vi "DOConfigureCustomaPattern.vi"(0 "object in":refnum<class "AD2_DO_SDK.lvclass">, 2 "?":T1={"DO Trigger"={"secRun(0=Cont)"=0.0, "secWait"=0.0, "cRepeat(0=inf)"=0, "Repeat Trigger"=FALSE, "TrigrSrc"=enum."trigrsrcNone"}, "CustomData"=[{"Data"=[FALSE, TRUE, FALSE, FALSE, FALSE, FALSE, FALSE, FALSE, FALSE, FALSE, FALSE, FALSE, FALSE, FALSE, FALSE, FALSE, FALSE, FALSE, FALSE, FALSE, FALSE, FALSE], "Freq"=1000.0, "#Bits"=100, "Enable"=FALSE, "IdleState"=0}, {"Data"=[TRUE, TRUE, TRUE, TRUE, TRUE, FALSE, FALSE, FALSE, FALSE, FALSE, FALSE, FALSE, FALSE, FALSE, FALSE, FALSE, FALSE, FALSE, FALSE, FALSE, FALSE, FALSE], "Freq"=1000.0, "#Bits"=100, "Enable"=FALSE, "IdleState"=0}, {"Data"=[], "Freq"=0.0, "#Bits"=0, "Enable"=FALSE, "IdleState"=0}, {"Data"=[FALSE, FALSE, FALSE, FALSE, FALSE, FALSE, FALSE, FALSE, FALSE, FALSE, FALSE, FALSE, FALSE, FALSE, FALSE, FALSE, FALSE, FALSE, FALSE, FALSE, FALSE, FALSE, FALSE], "Freq"=0.0, "#Bits"=0, "Enable"=FALSE, "IdleState"=0}, {"Data"=[], "Freq"=0.0, "#Bits"=0, "Enable"=FALSE, "IdleState"=0}, {"Data"=[], "Freq"=0.0, "#Bits"=0, "Enable"=FALSE, "IdleState"=0}, {"Data"=[], "Freq"=0.0, "#Bits"=0, "Enable"=FALSE, "IdleState"=0}, {"Data"=[], "Freq"=0.0, "#Bits"=0, "Enable"=FALSE, "IdleState"=0}, {"Data"=[], "Freq"=0.0, "#Bits"=0, "Enable"=FALSE, "IdleState"=0}, {"Data"=[], "Freq"=0.0, "#Bits"=0, "Enable"=FALSE, "IdleState"=0}, {"Data"=[], "Freq"=0.0, "#Bits"=0, "Enable"=FALSE, "IdleState"=0}, {"Data"=[], "Freq"=0.0, "#Bits"=0, "Enable"=FALSE, "IdleState"=0}, {"Data"=[], "Freq"=0.0, "#Bits"=0, "Enable"=FALSE, "IdleState"=0}, {"Data"=[], "Freq"=0.0, "#Bits"=0, "Enable"=FALSE, "IdleState"=0}, {"Data"=[], "Freq"=0.0, "#Bits"=0, "Enable"=FALSE, "IdleState"=0}, {"Data"=[FALSE, FALSE, FALSE, FALSE, FALSE, FALSE, FALSE, FALSE, FALSE, FALSE, FALSE, FALSE, FALSE, FALSE, FALSE, FALSE, FALSE, FALSE, FALSE, FALSE, FALSE, FALSE, FALSE], "Freq"=0.0, "#Bits"=0, "Enable"=FALSE, "IdleState"=0}, {"Data"=[FALSE, FALSE, FALSE, FALSE, FALSE, FALSE, FALSE, FALSE, FALSE, FALSE, FALSE, FALSE, FALSE, FALSE, FALSE, FALSE, FALSE, FALSE, FALSE, FALSE, FALSE, FALSE, FALSE], "Freq"=0.0, "#Bits"=0, "Enable"=FALSE, "IdleState"=0}]}, 5 "error in (no error)":errorcluster) -> (14 "object out":refnum<class "AD2_DO_SDK.lvclass">, 19 "error out":errorcluster)   [LabVIEW 2021, in "AD2_DO_SDK.lvclass"]
uses:
  AD2_DO_SDK.lvclass
  DOConfigureCustomData.ctl
  DOTrigger.ctl
  AD2_WFG_SDK_class/AD2TriggerSources.ctl
  DOCustomData.ctl
  AD2_DO_SDK.lvclass/AD2_DO_SDK.ctl
  Olasdwf/Olasdwf.lvlib
  AD2_SDK_class/AD2_SDK.lvclass
panel:
  out "In Range?":bool
  out "pcountOfBitsMax out":u32
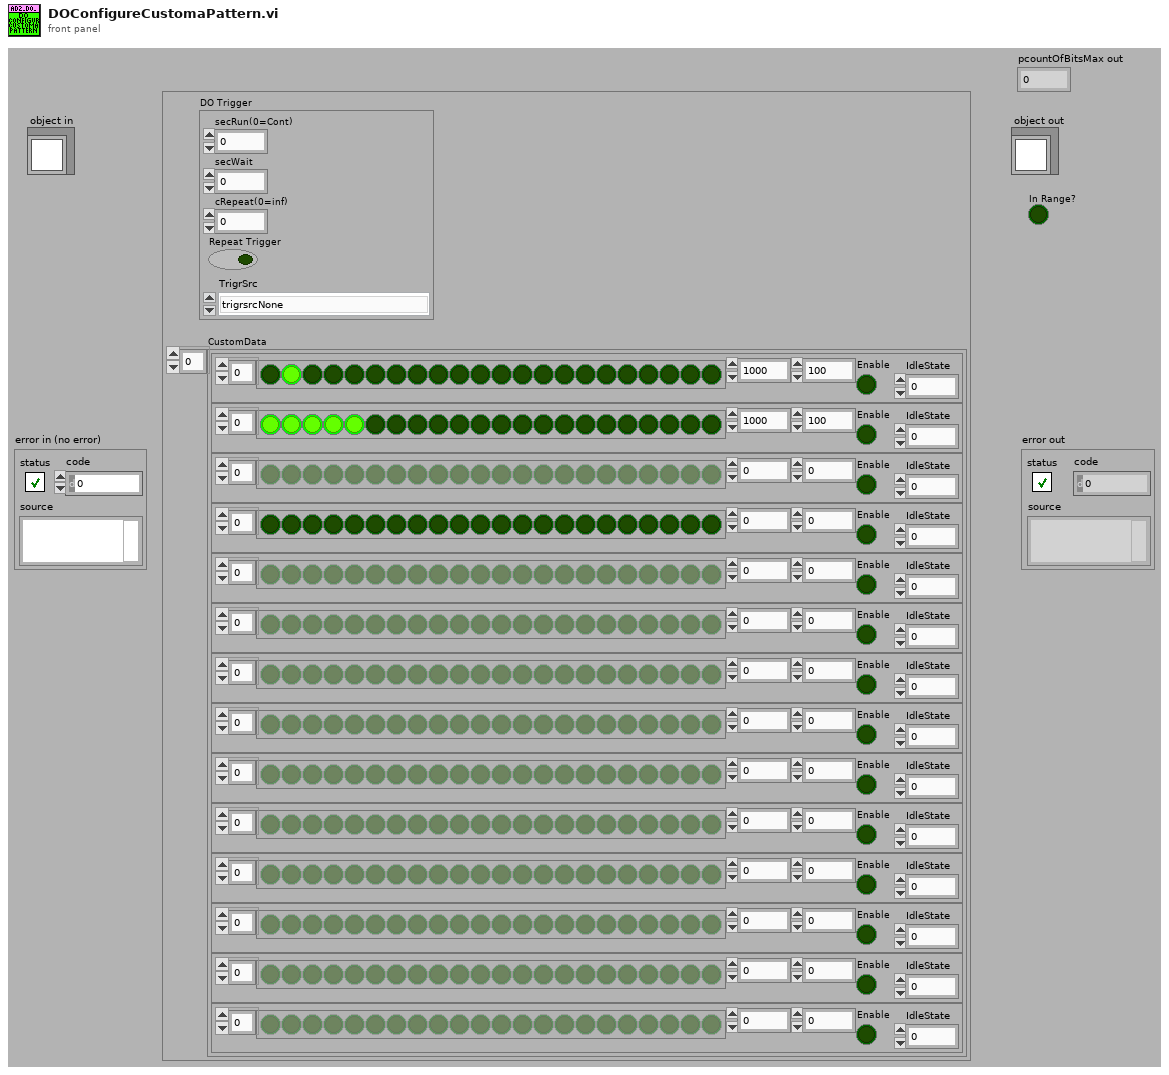
[diagram p1: front panel]
types:
  T1 = typedef "DOConfigureCustomData.ctl" = cluster{"DO Trigger":T2, "CustomData":T4}
  T2 = typedef "AD2_DO_SDK.lvclass/DOTrigger.ctl" = cluster{"secRun(0=Cont)":dbl, "secWait":dbl, "cRepeat(0=inf)":i32, "Repeat Trigger":bool, "TrigrSrc":T3}
  T3 = typedef "AD2_SDK.lvclass/AD2TriggerSources.ctl" = enum8{"trigrsrcNone", "trigsrcPC", "trigsrcDetectorAnalogIn", "trigsrcDetectorDigitalIn", "trigsrcAnalogIn", "trigsrcDigitalIn", "trigsrcDigitalOut", "trigsrcAnalogOut1", "trigsrcAnalogOut2", "trigsrcAnalogOut3", "trigsrcAnalogOut4", "trigsrcExternal1", "trigsrcExternal2", "trigsrcExternal3", "trigsrcExternal4", ""}
  T4 = typedef "AD2_DO_SDK.lvclass/DOCustomData.ctl" = cluster{"Data":bool[], "Freq":dbl, "#Bits":u32, "Enable":bool, "IdleState":u16}[]
  T5 = cluster{"NoHighBits":u32, "NoLowBits":u32, "NoInitialBits":u32, "Start High":bool}
  T6 = typedef "AD2_DO_SDK.lvclass/DOSingleCh.ctl" = cluster{"Ch Index":i32, "Enable":bool, "Clock DIvider":u32, "Type":i32, "DigitalOutOutput":u16, "IdleState":u16, "CounterData":cluster{"NoHighBits":u32, "NoLowBits":u32, "NoInitialBits":u32, "Start High":bool}, "Custom Data":cluster{"countOfBits":u32, "rgBits":u8[]}}
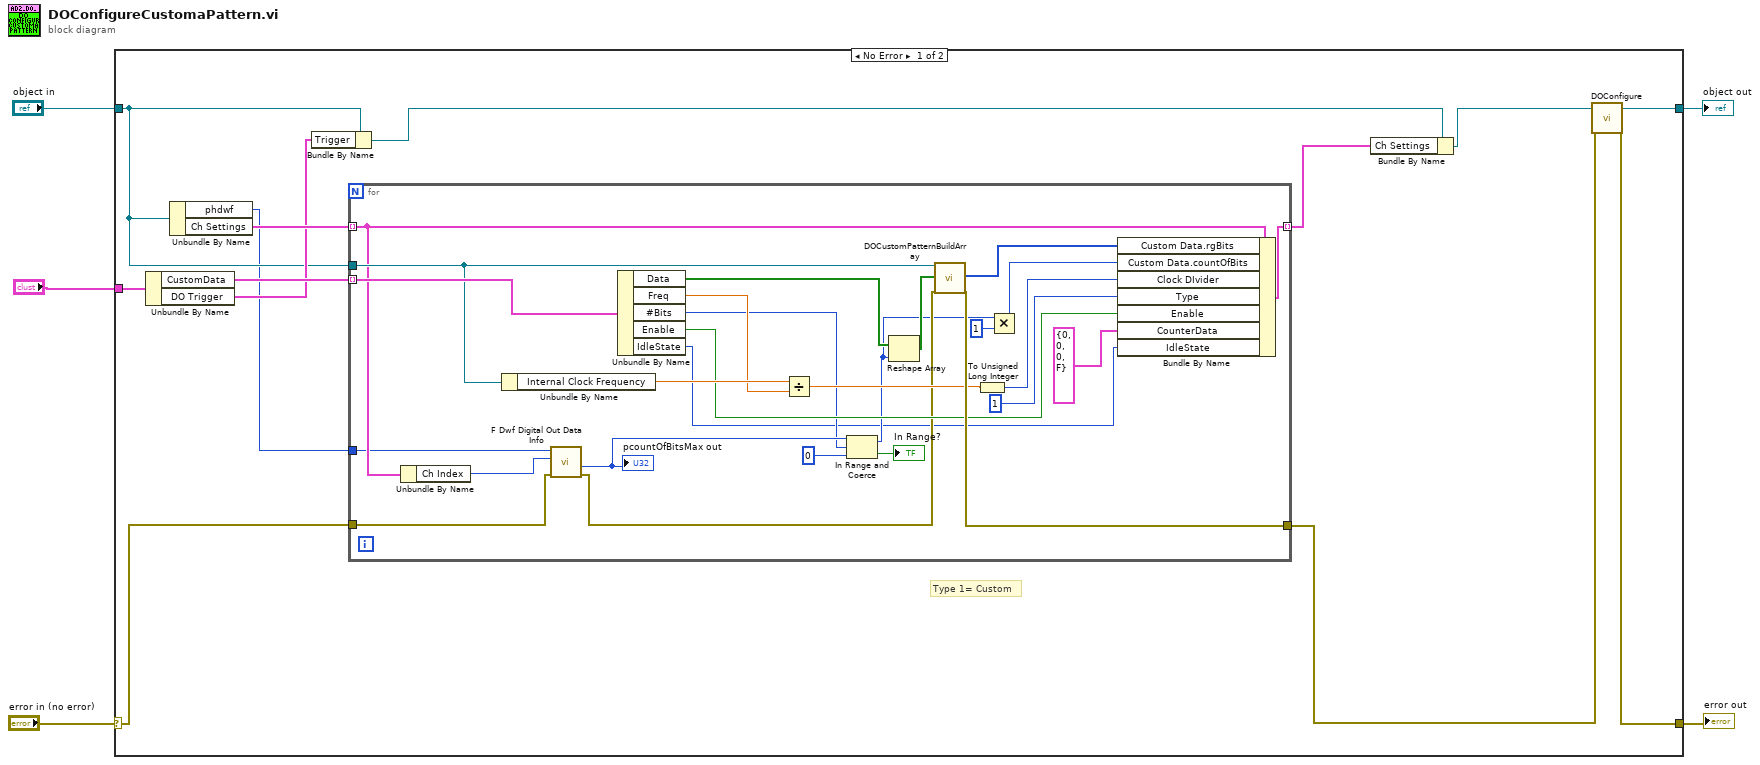
[diagram p0: block diagram]
diagram:
  n1 = case shown="No Error" "error in (no error)" {
    selector: "error in (no error)" -> [w10 w47]
    tunnel: [w18 w47] -> w4
    tunnel: [w17 w46] -> w2
    tunnel: "object in" -> [w7 w46]
    tunnel: "?" -> [w12 _]
    frame No Error {
      # "Type 1= Custom"
      n2 = Unbundle By Name(w12) -> ("CustomData"=w11:T4, "DO Trigger"=w9:T2)
      n3 = Unbundle By Name(w7) -> ("phdwf"=w6:i32, "Ch Settings"=w16:T6[])
      n4 = Bundle By Name(cluster=w7, "Trigger"=w9) -> (w8:refnum<class "AD2_DO_SDK.lvclass">)
      n5 = for {
        tunnel: w16 -> [w29] mode=indexing
        tunnel: [w45] -> w14 mode=indexing
        tunnel: w11 -> [w38] mode=indexing
        tunnel: w10 -> [w25]
        tunnel: [w43] -> w13
        tunnel: w7 -> [w37]
        tunnel: w6 -> [w28]
        n6 = Unbundle By Name(w29) -> ("Ch Index"=w27:i32)
        n7 = Unbundle By Name(w37) -> ("Internal Clock Frequency"=w36:dbl)
        n8 = call "F Dwf Digital Out Data Info.vi"("error in (no error)"=w25, "idxChannel"=w27, "hdwf"=w28) -> ("error out"=w26:errorcluster, "pcountOfBitsMax out"=w24:u32)  [unwired: 6 in, 1 out]
        "pcountOfBitsMax out" <- w24
        n9 = Unbundle By Name(w38) -> ("Data"=w42:bool[], "Freq"=w35:dbl, "#Bits"=w21:u32, "Enable"=w31:bool, "IdleState"=w19:u16)
        n10 = Divide(x=w36, y=w35) -> (x/y=w34:dbl)
        n11 = In Range and Coerce(upper limit=w24, x=w21, lower limit=u32 0) -> (coerced(x)=w20:u32, In Range?=→"In Range?":bool)
        n12 = Reshape Array(w42, w20) -> (w41:bool[])
        n13 = call-dynamic "DOCustomPatternBuildArray.vi"("object in"=w37, "Data"=w41, "error in (no error)"=w26) -> ("Array"=w44:u8[], "error out"=w43:errorcluster)  [unwired: 14 in, 1 out]
        n14 = To Unsigned Long Integer(number=w34) -> (unsigned 32bit integer=w33:u32)
        n15 = Multiply(x=w20, y=u32 1) -> (x*y=w39:u32)
        n16 = Bundle By Name(cluster=w29, "Custom Data.rgBits"=w44, "Custom Data.countOfBits"=w39, "Clock DIvider"=w33, "Type"=1, "Enable"=w31, "CounterData"=T5 {"NoHighBits"=0, "NoLowBits"=0, "NoInitialBits"=0, "Start High"=FALSE}, "IdleState"=w19) -> (w45:T6)
      }
      n17 = Bundle By Name(cluster=w8, "Ch Settings"=w14) -> (w15:refnum<class "AD2_DO_SDK.lvclass">)
      n18 = call-dynamic "DOConfigure.vi"("object in"=w15, "error in (no error)"=w13) -> ("object out"=w17:refnum<class "AD2_DO_SDK.lvclass">, "error out"=w18:errorcluster)  [unwired: 16 in]
    }
    frame Error {
    }
  }
  "error out" <- w4
  "object out" <- w2
